vi "Write Field - U32 Array.vi"(7 "field name":string, 8 "error in":errorcluster, 10 "value":u32[](array[numeric]), 11 "PV Data in":refnum<class "PV Data.lvclass">) -> (0 "error out":errorcluster, 2 "value out":u32[](array[numeric]), 3 "PV Data out":refnum<class "PV Data.lvclass">)   [LabVIEW 2020, in "PV Access.lvlib" / "PV Data.lvlib" / "PV Data.lvclass"]
uses:
  PV Data.lvclass
  PV Access.lvlib
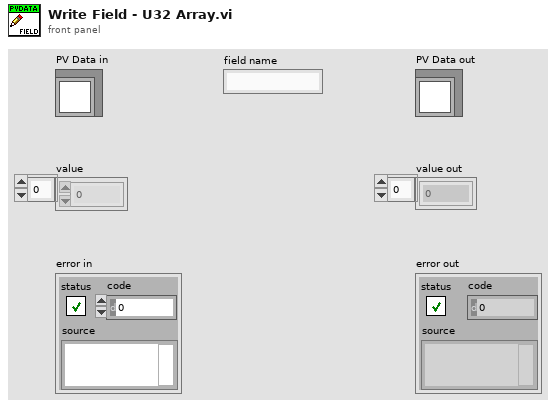
[diagram p1: front panel]
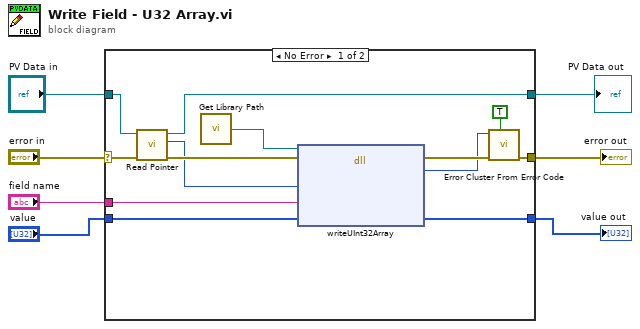
[diagram p0: block diagram]
diagram:
  n1 = case shown="No Error" "error in" {
    selector: "error in" -> [w12 w23]
    tunnel: [w14 w23] -> w7
    tunnel: "value" -> [w20 w22]
    tunnel: [w19 w22] -> w4
    tunnel: [w10 w21] -> w2
    tunnel: "PV Data in" -> [w13 w21]
    tunnel: "field name" -> [w8 _]
    frame No Error {
      n2 = call-dynamic "Read Pointer.vi"("error in (no error)"=w12, "Pointer Base in"=w13) -> ("error out"=w11:errorcluster, "Pointer"=w9:i64, "Pointer Base out"=w10:refnum<class "PV Data.lvclass">)  [unwired: 7 in]
      n3 = call "Get Library Path.vi"() -> ("Path"=w18:path)  [unwired: 1 in]
      n4 = dll-call lib="?" fn="writeUInt32Array"(path in=w18, error in=w11, "value"=w9, "field_name"=w8, "new_value"=w20) -> (error out=w16:errorcluster, "err_code"=w15:i32, "new_value"=w19:u32[])  [unwired: 3 in, 1 out]
      n5 = call <vilib>:"Error Cluster From Error Code.vi"("show call chain? (False)"=TRUE, "error in (no error)"=w16, "error code (0)"=w15) -> ("error out"=w14:errorcluster)  [unwired: 6 in]
    }
    frame Error {
    }
  }
  "error out" <- w7
  "value out" <- w4
  "PV Data out" <- w2
